vi "Eval y=f(x) Optimal Step.vi"(4 "number of points":u32=10, 5 "formula":string, 6 "end":dbl=1.0 format="%.2f", 7 "start":dbl format="%.2f", 8 "epsilon":dbl=0.05 min=1e-18 format="%.2f") -> (0 "error":i32, 1 "ticks":u32, 2 "Y Values":dbl[](array[numeric]) format="%.2f", 3 "X Values":dbl[](array[numeric]) format="%.2f")   [LabVIEW 2018, in "NI_Gmath.lvlib"]
doc: "Calculates the values of a more complex 1D function given by a <B>formula</B>."
uses:
  NI_Gmath.lvlib
panel:
  # "Example:\n\n number of points: 100 \n epsilon: 0.05\n start: 0.0\n end: 1.0\n formula: sin(t*t)+t"
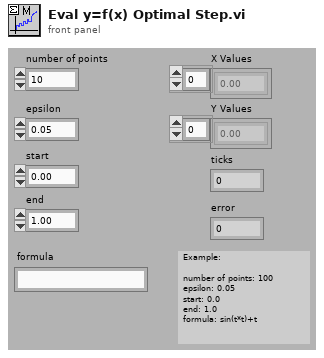
[diagram p1: front panel]
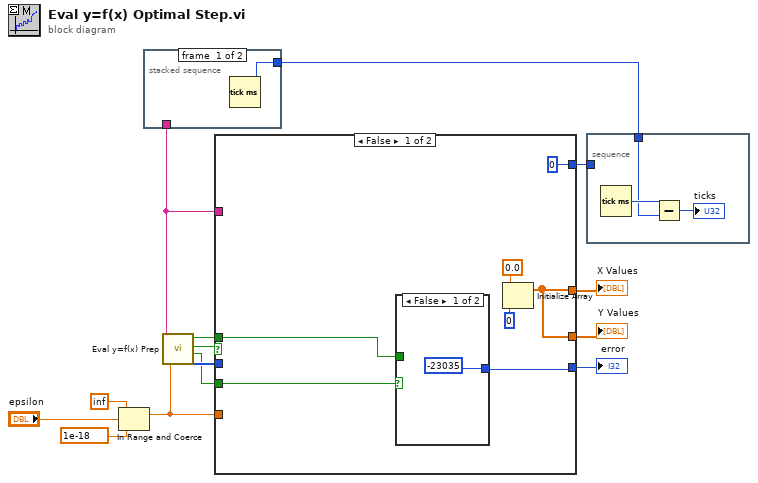
[diagram p0: block diagram]
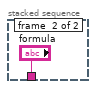
[diagram p2: hidden frame]
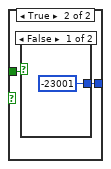
[diagram p3: hidden frame]
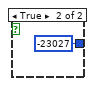
[diagram p4: hidden frame]
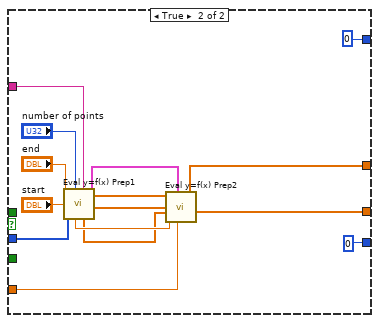
[diagram p5: hidden frame]
diagram:
  n1 = In Range and Coerce(upper limit=inf, x="epsilon", lower limit=1e-18) -> (coerced(x)=w2:dbl)  [unwired: 1 out]
  n2 = stacked-sequence {
    tunnel: [w15 _] -> w13
    tunnel: [_ "formula"] -> w5
    frame #0 {
      n3 = Tick Count (ms)() -> (millisecond timer value=w15:u32)
    }
    frame #1 {
    }
  }
  n4 = call "Eval y=f(x) Prep.vi"("formula"=w5, "epsilon"=w2) -> ("error (formula)"=w8:bool, "error (general)"=w7:bool, "error (epsilon)"=w6:bool, "List of variables"=w14:i32[])
  n5 = case shown="False" w7 {
    tunnel: w5 -> [_ w43]
    tunnel: w14 -> [_ w42]
    tunnel: [w21 w34] -> w12
    tunnel: [w21 w33] -> w11
    tunnel: [0 0] -> w10
    tunnel: [w19 0] -> w9
    tunnel: w8 -> [w18 _]
    tunnel: w2 -> [_ w30]
    tunnel: w6 -> [w17 _]
    frame False {
      n6 = case shown="False" w17 {
        tunnel: w18 -> [_ w26]
        tunnel: [-23035 w25] -> w19
        frame False {
        }
        frame True {
          n7 = case shown="False" w26 {
            tunnel: [-23001 -23027] -> w25
            frame False {
            }
            frame True {
            }
          }
        }
      }
      n8 = Initialize Array(0.0, 0) -> (w21:dbl[])
    }
    frame True {
      n9 = call "Eval y=f(x) Prep1.vi"("end"="end", "number of points"="number of points", "start"="start", "List of variables"=w42, "formula"=w43) -> ("random summand"=w39:dbl, "Parsed Formula"=w29:cluster{"Table":i32[][], "Y Values":dbl[]}, "points"=w37:dbl[], "points II"=w36:dbl[], "points I"=w35:dbl[])
      n10 = call "Eval y=f(x) Prep2 .vi"("epsilon"=w30, "Parsed Formula"=w29, "random summand"=w39, "points II in"=w36, "points I in"=w35, "points in"=w37) -> ("points I out"=w33:dbl[], "points out"=w34:dbl[])
    }
  }
  "X Values" <- w12
  "Y Values" <- w11
  "error" <- w9
  n11 = stacked-sequence {
    tunnel: w13 -> [w44]
    tunnel: w10 -> [_]
    frame #0 {
      n12 = Tick Count (ms)() -> (millisecond timer value=w45:u32)
      n13 = Subtract(x=w45, y=w44) -> (x-y=→"ticks":u32)
    }
  }
